vi "Impedance tube v0.1.vi"() -> ()   [LabVIEW 2021]
uses:
  <vilib>/Analysis/2dsp.llb/Real FFT.vi
  <vilib>/Analysis/NI_AALPro.lvlib
panel:
  out "Transfer function":dbl[](graph)
  out "MIC 2":dynamicdata(graph)
  out "FFT2":dbl[](graph)
  in  "FFT size 2":i32=-1
  out "MIC 2":dbl
  out "FFT1":dbl[](graph)
  out "MIC 1":dynamicdata(graph)
  in  "FFT size":i32=-1
  out "MIC 1":dbl
  in  "stop (F)":bool
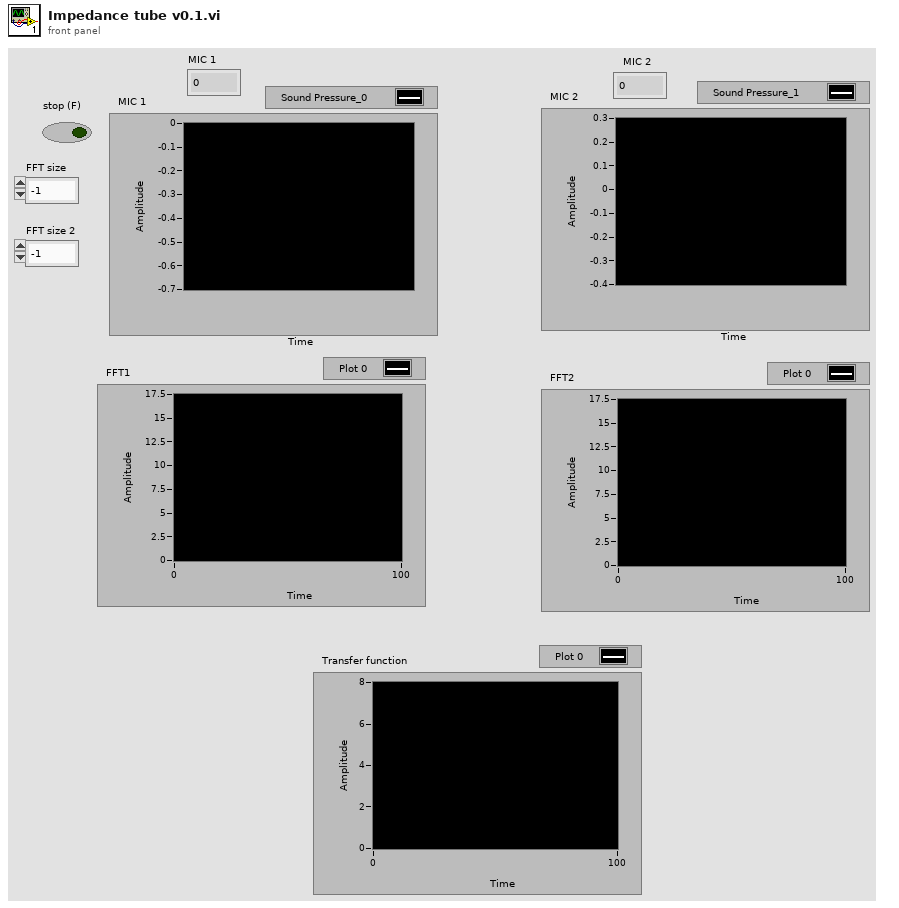
[diagram p1: front panel]
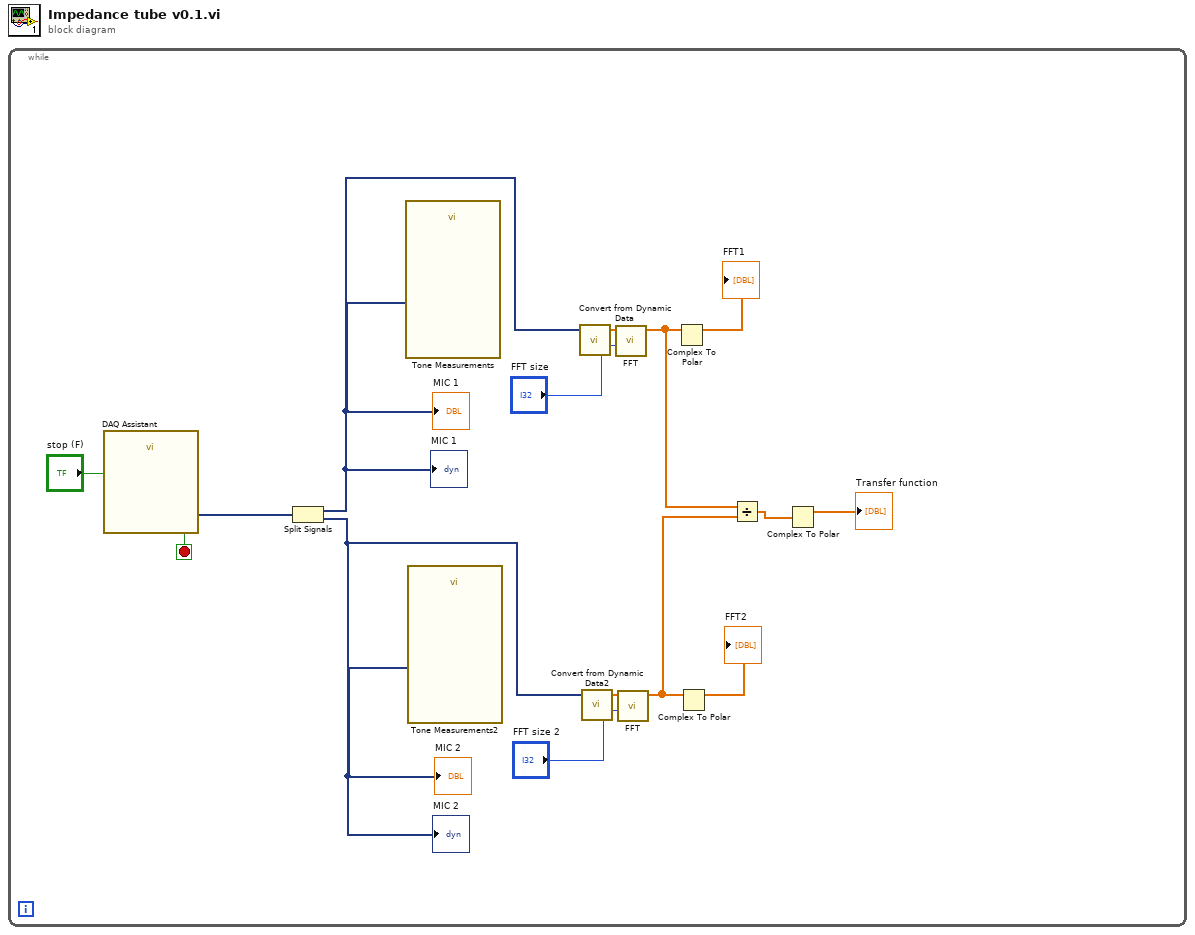
[diagram p0: block diagram]
diagram:
  n1 = while {
    stop <- w14 stop-if-true
    n2 = call "DAQ Assistant"("stop (F)"="stop (F)") -> ("data"=w10:dynamicdata, "stopped"=w14:bool)  [unwired: 15 in, 2 out]
    n3 = Split Signals(w10) -> (w6:dynamicdata, w3:dynamicdata)  [unwired: 2 in]
    "MIC 1" <- w6
    "MIC 1" <- w6
    "MIC 2" <- w3
    "MIC 2" <- w3
    n4 = call "Tone Measurements"("Signals"=w6) -> ()  [unwired: 8 in, 3 out]
    n5 = call "Tone Measurements2"("Signals"=w3) -> ()  [unwired: 8 in, 3 out]
    n6 = call "Convert from Dynamic Data"("Dynamic Data Type"=w6) -> ("Array"=w12:dbl[])  [unwired: 3 in]
    n7 = call "Convert from Dynamic Data2"("Dynamic Data Type"=w3) -> ("Array"=w8:dbl[])  [unwired: 3 in]
    n8 = call-poly <vilib>:"FFT.vi"("FFT size"="FFT size", "X"=w12) -> ("FFT {X}"=w5:cdb[])  [unwired: 8 in, 1 out]
    n9 = call-poly <vilib>:"FFT.vi"("FFT size"="FFT size 2", "X"=w8) -> ("FFT {X}"=w4:cdb[])  [unwired: 8 in, 1 out]
    n10 = Complex To Polar(r * e^(i*theta)=w5) -> (r=→"FFT1":dbl[])  [unwired: 1 out]
    n11 = Complex To Polar(r * e^(i*theta)=w4) -> (r=→"FFT2":dbl[])  [unwired: 1 out]
    n12 = Divide(x=w5, y=w4) -> (x/y=w2:cdb[])
    n13 = Complex To Polar(r * e^(i*theta)=w2) -> (r=→"Transfer function":dbl[])  [unwired: 1 out]
  }
